vi "LakeShore Curve Manager.vi"(0 "VISA session":refnum<visa-resource-name>) -> ()   [LabVIEW 2019]
doc: "This VI will poll the specified GPIB address for a LakeShore Temperature Controller or Resistance Bridge, determine the model number of the device, and run the appropriate Curve Manager.\n\nJonathan Billings <billings@magnet.fsu.edu> NHMFL-FSU, April 2010"
panel:
  # "Select the GPIB Address for the Temperature Controler,\nthen run this VI."
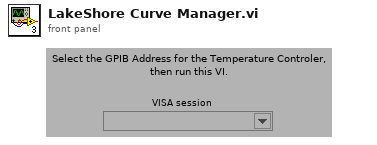
[diagram p1: front panel]
types:
  T1 = enum32{"Invalid", "Standard", "Closed", "Hidden", "Minimized", "Maximized"}
  T2 = enum32{"Bad", "Idle", "Run top level", "Running"}
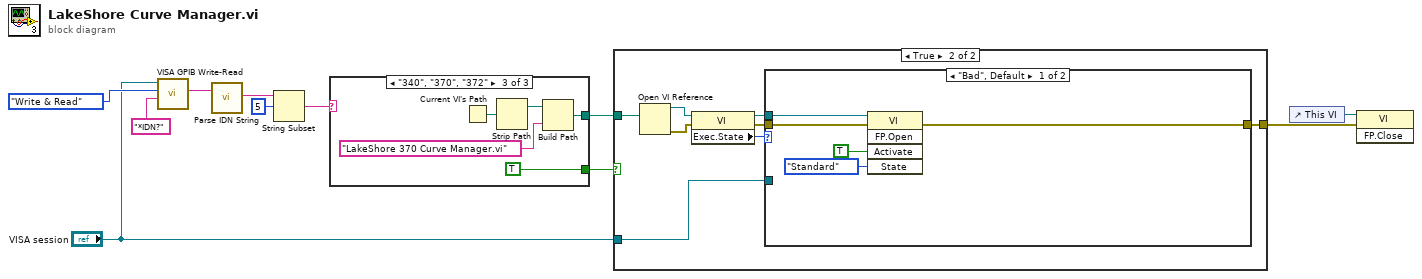
[diagram p0: block diagram]
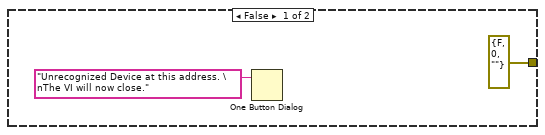
[diagram p2: hidden frame]
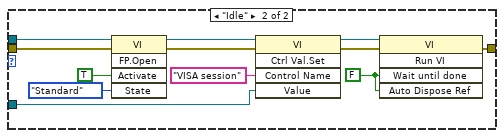
[diagram p3: hidden frame]
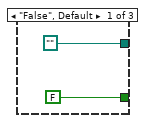
[diagram p4: hidden frame]
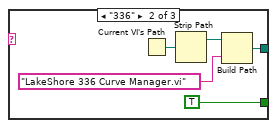
[diagram p5: hidden frame]
diagram:
  n1 = call "VISA GPIB Write-Read.vi"("Command"="*IDN?" ("String to Write"), "Action"=enum16{"Write", "Read", "Write & Read"}."Write & Read", "VISA resource name"="VISA session") -> ("String Returned"=w9:string)  [unwired: 5 in, 3 out]
  n2 = call "Parse IDN String.vi"("IDN String"=w9) -> ("Model"=w5:string)  [unwired: 1 in, 4 out]
  n3 = String Subset(string=w5, offset (0)=5) -> (substring=w4:string)  [unwired: 1 in]
  n4 = case shown="\"340\", \"370\", \"372\"" w4 {
    tunnel: [path "" w15 w20] -> w11
    tunnel: [FALSE TRUE TRUE] -> w3
    frame "False", Default {
    }
    frame "336" {
      n5 = Current VI's Path() -> (path=w17:path)
      n6 = Strip Path(path=w17) -> (stripped path=w16:path)  [unwired: 1 out]
      n7 = Build Path(base path=w16, name or relative path="LakeShore 336 Curve Manager.vi") -> (appended path=w15:path)
    }
    frame "340", "370", "372" {
      n8 = Current VI's Path() -> (path=w22:path)
      n9 = Strip Path(path=w22) -> (stripped path=w21:path)  [unwired: 1 out]
      n10 = Build Path(base path=w21, name or relative path="LakeShore 370 Curve Manager.vi") -> (appended path=w20:path)
    }
  }
  n11 = case shown="True" w3 {
    tunnel: w11 -> [_ w33]
    tunnel: "VISA session" -> [_ w29]
    tunnel: [errorcluster {"status"=FALSE, "code"=0, "source"=""} ("error out") w27] -> w1
    frame False {
      n12 = One Button Dialog(message="Unrecognized Device at this address. \nThe VI will now close.") -> ()  [unwired: 1 in, 1 out]
    }
    frame True {
      n13 = Open VI Reference(vi path=w33) -> (vi reference=w28:refnum<vi>, error out=w32:errorcluster)  [unwired: 5 in]
      n14 = property class="VI"(reference=w28, error in=w32) -> (reference out=w30:refnum<vi>, error out=w31:errorcluster, "Exec.State"=w26:T2)
      n15 = case shown="\"Bad\", Default" w26 {
        tunnel: w31 -> [w38 w50]
        tunnel: w30 -> [w37 w49]
        tunnel: w29 -> [_ w48]
        tunnel: [w34 w39] -> w27
        frame "Bad", Default {
          n16 = invoke class="VI" method="FP.Open"(reference=w37, error in=w38, "Activate"=TRUE ("Activate?"), "State"=T1."Standard") -> (error out=w34:errorcluster)  [unwired: 1 in, 4 out]
        }
        frame "Idle" {
          w40 = FALSE ("Wait Until Done")
          n17 = invoke class="VI" method="FP.Open"(reference=w49, error in=w50, "Activate"=TRUE ("Activate?"), "State"=T1."Standard") -> (reference out=w45:refnum<vi>, error out=w43:errorcluster)  [unwired: 1 in, 3 out]
          n18 = invoke class="VI" method="Ctrl Val.Set"(reference=w45, error in=w43, "Control Name"="VISA session", "Value"=w48) -> (reference out=w42:refnum<vi>, error out=w41:errorcluster)  [unwired: 1 in, 3 out]
          n19 = invoke class="VI" method="Run VI"(reference=w42, error in=w41, "Wait until done"=w40, "Auto Dispose Ref"=w40) -> (error out=w39:errorcluster)  [unwired: 1 in, 4 out]
        }
      }
    }
  }
  n20 = control-ref of="This VI"() -> (w2:refnum<vi>)
  n21 = invoke class="VI" method="FP.Close"(reference=w2, error in=w1) -> ()  [unwired: 1 in, 3 out]
